vi "CustomPID_v1.4.vi"(0 "MaxOutput":dbl, 1 "MinOutput":dbl, 2 "Epsilon":dbl, 3 "pK":dbl, 4 "dK":dbl, 5 "iK":dbl, 6 "Process Variable":dbl, 7 "Reinit":bool, 9 "Shutoff Time (ms)":u32, 12 "Setpoint":dbl) -> (16 "Output":dbl, 18 "CurrentError":dbl)   [LabVIEW 2014]
panel:
  out "CurrentIntegral":dbl
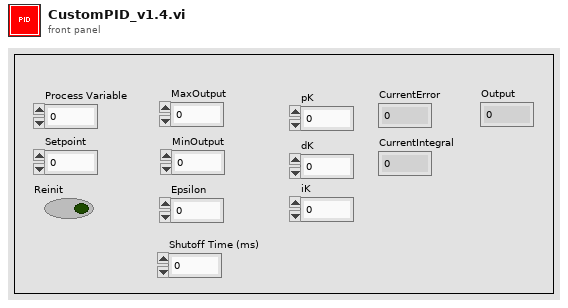
[diagram p1: front panel]
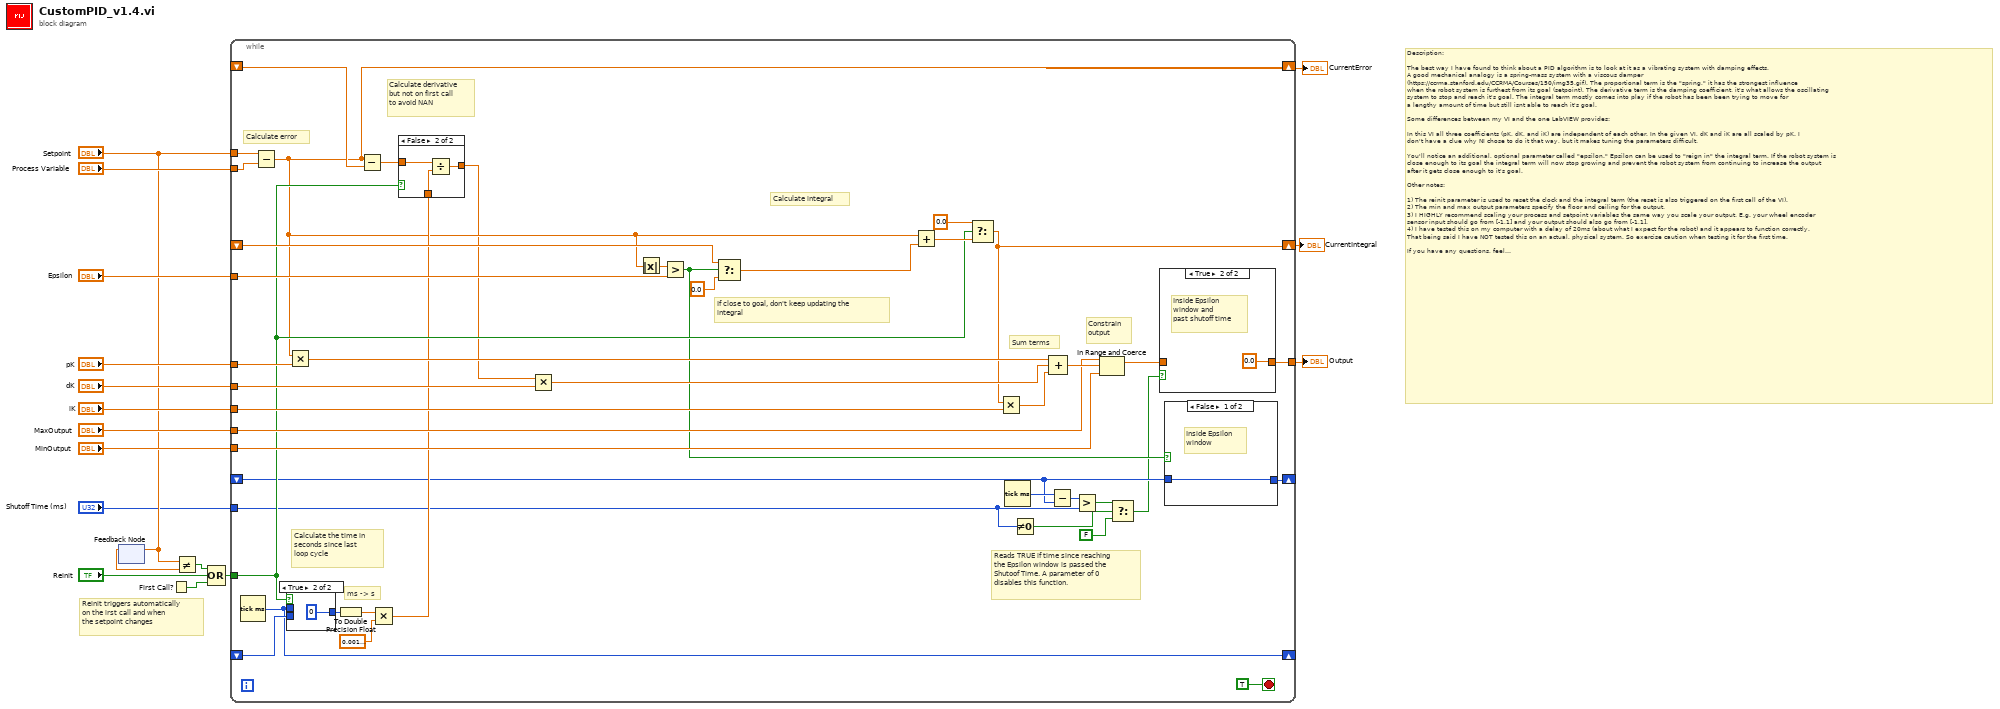
[diagram p0: block diagram]
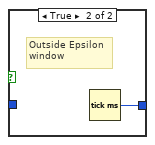
[diagram p2: hidden frame]
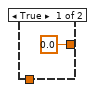
[diagram p4: hidden frame]
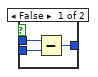
[diagram p5: hidden frame]
diagram:
  # "Reinit triggers automatically\non the irst call and when \nthe setpoint changes"
  # "Description:\n\nThe best way I have found to think about a PID algorithm is to look at it as a vibrating system with damping effects.\nA good mechanical analogy is a spring-mass system with a viscous damper \n(https://ccrma.stanford.edu/CCRMA/Courses/150/img35.gif). The proportional term is the \"spring,\" it has the strongest influence\nwhen the robot system is furthest from its goal (setpoint). The derivative term is the damping coefficient, it's what allows the oscillating\nsystem to stop and reach it's goal. The integral term mostly comes into play if the robot has been been trying to move for \na lengthy amount of time but still isnt able to reach it's goal.\n\nSome differences between my VI and the one LabVIEW provides:\n\nIn this VI all three coefficients (pK, dK, and iK) are independent of each other. In the given VI, dK and iK are all scaled by pK. I\ndon't have a clue why NI chose to do it that way, but it makes tuning the parameters difficult. \n\nYou'll notice an additional, optional parameter called \"epsilon.\" Epsilon can be used to \"reign in\" the integral term. If the robot system is \nclose enough to its goal the integral term will now stop growing and prevent the robot system from continuing to increase the output\nafter it gets close enough to it's goal.\n\nOther notes:\n\n1) The reinit parameter is used to reset the clock and the integral term (the reset is also triggered on the first call of the VI).\n2) The min and max output parameters specify the floor and ceiling for the output.\n3) I HIGHLY recommend scaling your process and setpoint variables the same way you scale your output. E.g. your wheel encoder \nsensor input should go from [-1,1] and your output should also go from [-1,1].\n4) I have tested this on my computer with a delay of 20ms (about what I expect for the robot) and it appears to function correctly.\nThat being said I have NOT tested this on an actual, physical system. So exercise caution when testing it for the first time.\n\nIf you have any questions, feel free to contact me,\n-Luke (lrscime@ufl.edu)"
  n1 = feedback #1() -> (w7:dbl)  [unwired: 1 in]
  n2 = feedback-in #1("Setpoint") -> ()
  n3 = First Call?() -> (First Call?: T/F=w4:bool)
  n4 = Not Equal?(x="Setpoint", y=w7) -> (x != y?=w2:bool)
  n5 = Compound Arithmetic op=OR(w2, "Reinit", w4) -> (w5:bool)
  n6 = while {
    tunnel: "Setpoint" -> [w59]
    shift-right: [w31] -> w11
    shift-left: _ -> [w58]
    shift-right: [w33] -> w10
    shift-left: _ -> [w50]
    tunnel: "pK" -> [w57]
    tunnel: "dK" -> [w56]
    tunnel: "iK" -> [w55]
    tunnel: "Epsilon" -> [w51]
    tunnel: [w28] -> w9
    tunnel: "MaxOutput" -> [w47]
    shift-right: [w44] -> _
    shift-left: _ -> [w45]
    tunnel: w5 -> [w36]
    tunnel: "MinOutput" -> [w40]
    tunnel: "Process Variable" -> [w32]
    shift-right: [w20] -> _
    shift-left: _ -> [w19]
    tunnel: "Shutoff Time (ms)" -> [w25]
    stop <- TRUE stop-if-true
    # "Reads TRUE if time since reaching\nthe Epsilon window is passed the \nShutoof Time. A parameter of 0 \ndisables this function."
    # "If close to goal, don't keep updating the\nintegral"
    # "Calculate the time in\nseconds since last\nloop cycle"
    # "Constrain\noutput"
    # "Sum terms"
    # "ms -> s"
    # "Calculate integral"
    # "Calculate derivative\nbut not on first call \nto avoid NAN"
    # "Calculate error"
    n7 = Tick Count (ms)() -> (millisecond timer value=w44:u32)
    n8 = Subtract(x=w59, y=w32) -> (x-y=w31:dbl)
    n9 = case shown="True" w36 {
      tunnel: [w71 u32 0] -> w42
      tunnel: w45 -> [w70 _]
      tunnel: w44 -> [w69 _]
      frame False {
        n10 = Subtract(x=w69, y=w70) -> (x-y=w71:u32)
      }
      frame True {
      }
    }
    n11 = Multiply(x=w31, y=w57) -> (x*y=w54:dbl)
    n12 = To Double Precision Float(number=w42) -> (double precision float=w41:dbl)
    n13 = Subtract(x=w31, y=w58) -> (x-y=w37:dbl)
    n14 = Multiply(x=w41, y=0.0010000000474974513) -> (x*y=w35:dbl)
    n15 = case shown="False" w36 {
      tunnel: [0.0 ("t") w68] -> w30
      tunnel: w37 -> [_ w67]
      tunnel: w35 -> [_ w66]
      frame True {
      }
      frame False {
        n16 = Divide(x=w67, y=w66) -> (x/y=w68:dbl)
      }
    }
    n17 = Multiply(x=w30, y=w56) -> (x*y=w53:dbl)
    n18 = Absolute Value(x=w31) -> (abs(x)=w34:dbl)
    n19 = Greater?(x=w34, y=w51) -> (0:w21:bool)
    n20 = Select(t=w50, s=w21, f=0.0) -> (s? t:f=w46:dbl)
    n21 = Add(x=w31, y=w46) -> (x+y=w39:dbl)
    n22 = Select(t=0.0, s=w36, f=w39) -> (s? t:f=w33:dbl)
    n23 = Multiply(x=w33, y=w55) -> (x*y=w52:dbl)
    n24 = Tick Count (ms)() -> (millisecond timer value=w27:u32)
    n25 = Not Equal To 0?(x=w25) -> (x != 0?=w23:bool)
    n26 = Compound Arithmetic op=ADD(w54, w53, w52) -> (w48:dbl)
    n27 = Subtract(x=w27, y=w19) -> (x-y=w26:u32)
    n28 = Greater?(x=w26, y=w25) -> (0:w24:bool)
    n29 = In Range and Coerce(upper limit=w47, x=w48, lower limit=w40) -> (coerced(x)=w29:dbl)  [unwired: 1 out]
    n30 = Select(t=w24, s=w23, f=FALSE) -> (s? t:f=w18:bool)
    n31 = case shown="True" w18 {
      tunnel: w29 -> [w63 _]
      tunnel: [w63 0.0 ("MaxOutput")] -> w28
      frame False {
        # "Outside Epsilon\nwindow or not \npast shutoff time"
      }
      frame True {
        # "Inside Epsilon\nwindow and  \npast shutoff time"
      }
    }
    n32 = case shown="False" w21 {
      tunnel: [w61 w62] -> w20
      tunnel: w19 -> [w61 _]
      frame False {
        # "Inside Epsilon\nwindow"
      }
      frame True {
        # "Outside Epsilon\nwindow"
        n33 = Tick Count (ms)() -> (millisecond timer value=w62:u32)
      }
    }
  }
  "CurrentError" <- w11
  "CurrentIntegral" <- w10
  "Output" <- w9
